vi "CallAbsoluteVI.vi"(1 "error in (no error)":errorcluster, 2 "VI Name":string="InstrumentName") -> (0 "error out":errorcluster)   [LabVIEW 2014]
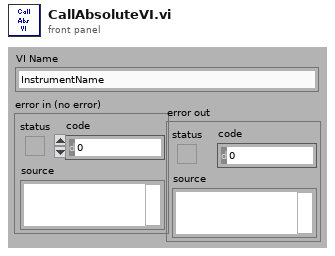
[diagram p1: front panel]
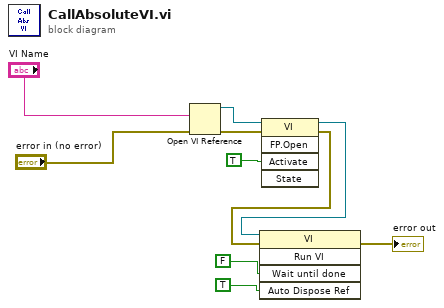
[diagram p0: block diagram]
diagram:
  n1 = Open VI Reference(vi path="VI Name", error in (no error)="error in (no error)") -> (vi reference=w5:refnum<vi>, error out=w8:errorcluster)  [unwired: 4 in]
  n2 = invoke class="VI" method="FP.Open"(reference=w5, error in=w8, "Activate"=TRUE ("Activate?")) -> (reference out=w7:refnum<vi>, error out=w6:errorcluster)  [unwired: 2 in, 3 out]
  n3 = invoke class="VI" method="Run VI"(reference=w7, error in=w6, "Wait until done"=FALSE, "Auto Dispose Ref"=TRUE) -> (error out=→"error out":errorcluster)  [unwired: 1 in, 4 out]
